vi "Waveform Amplitude Test.vi"(4 "EndRecordMask":i32, 6 "InitialRecordMask":i32, 8 "Lower Constant":dbl, 9 "Upper Constant":dbl=0.001, 10 "Channels to Exclude":string[](array[string]), 11 "Data In":waveform(dbl)[](array[waveform])) -> (1 "Within Limits":bool caption="Passed", 2 "Excluded Channels":waveform(dbl)[](array[waveform]), 3 "Included Channels":waveform(dbl)[](array[waveform]))   [LabVIEW 2019, in "Variant Parser.lvlib" / "WaveformProcessor.lvclass"]
doc: "This routine will look for violations of absolute max and min amplitudes.\nData In: Array of Labview Analog Waveforms to process\nChannels to exclude: Array if channels to ignore testing\nUpper Constant: Upper Amplitude limit\nLower Constant: Lower Amplitude limit\nInitial Record Mask - ignore number of records from t0\nFinal record mask - ignore number of data points from tf"
uses:
  Library/WaveformProcessor.lvclass
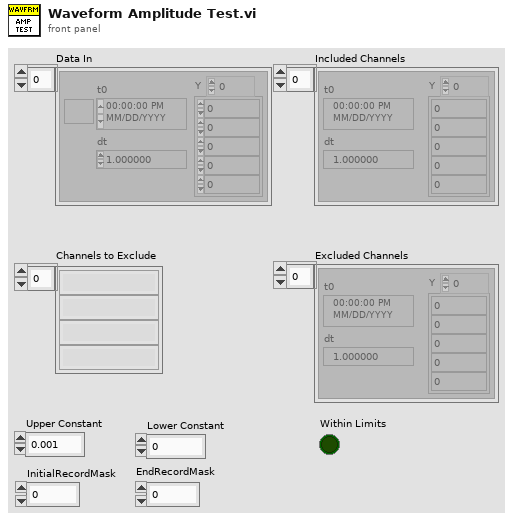
[diagram p1: front panel]
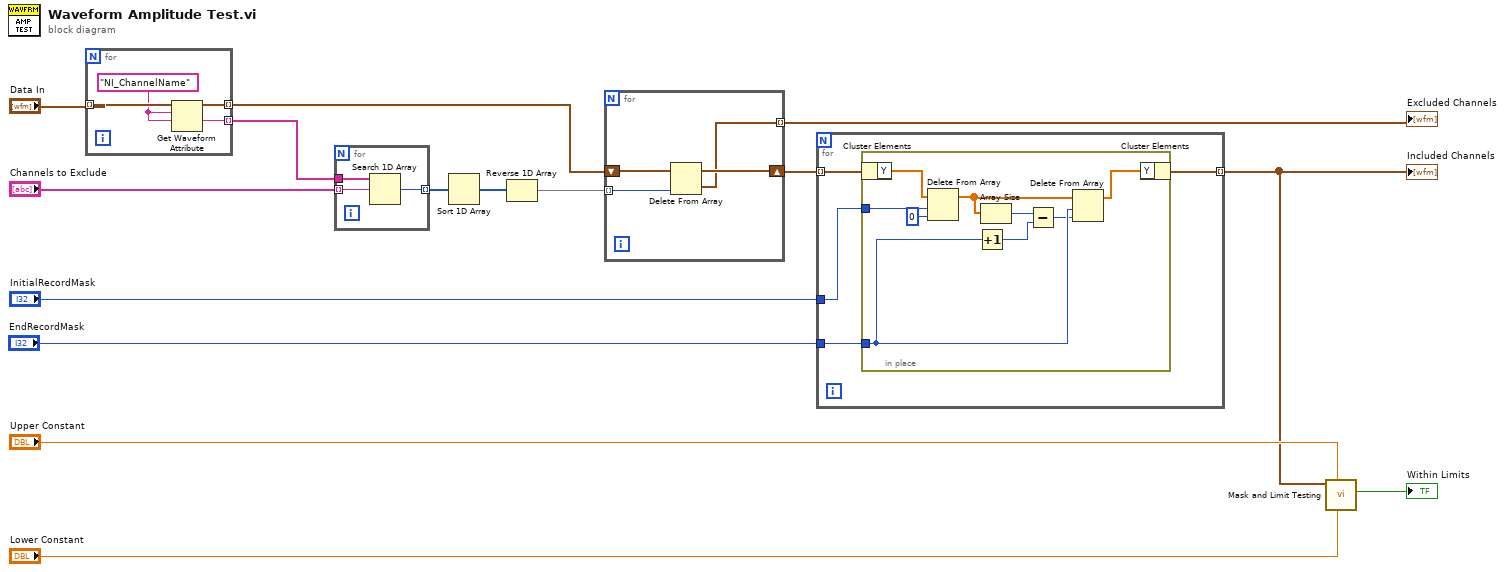
[diagram p0: block diagram]
diagram:
  n1 = for {
    tunnel: [w17] -> w14 mode=indexing
    tunnel: [w16] -> w10 mode=indexing
    tunnel: "Data In" -> [w19] mode=indexing
    w18 = "NI_ChannelName" ("name")
    n2 = Get Waveform Attribute(5:w18, 6:w18, 7:w19) -> (1:w16:string, 3:w17:waveform(dbl))  [unwired: 1 in, 2 out]
  }
  n3 = for {
    tunnel: "Channels to Exclude" -> [w22] mode=indexing
    tunnel: w10 -> [w21]
    tunnel: [w20] -> w11 mode=indexing
    n4 = Search 1D Array(1D array=w21, element=w22) -> (index of element=w20:i32)  [unwired: 1 in]
  }
  n5 = Sort 1D Array(array=w11) -> (sorted array=w12:i32[])
  n6 = Reverse 1D Array(array=w12) -> (reversed array=w13:i32[])
  n7 = for {
    tunnel: w13 -> [w24] mode=indexing
    shift-right: [w25] -> w4
    shift-left: w14 -> [w26]
    tunnel: [w23] -> w15 mode=indexing
    n8 = Delete From Array(array=w26, index=w24) -> (deleted portion=w23:waveform(dbl), array with subset deleted=w25:waveform(dbl)[])  [unwired: 1 in]
  }
  "Excluded Channels" <- w15
  n9 = for {
    tunnel: w4 -> [w30] mode=indexing
    tunnel: [w29] -> w3 mode=indexing
    tunnel: "InitialRecordMask" -> [w28]
    tunnel: "EndRecordMask" -> [w27]
    n10 = in-place {
      in-place-border: w28 -> [w34]
      in-place-border: w27 -> [w32]
      n11 = in-place-cluster #1(w30) -> ("Y"=w39:dbl[])
      n12 = Delete From Array(array=w39, length=w34, index=0) -> (array with subset deleted=w37:dbl[])  [unwired: 1 out]
      n13 = Increment(x=w32) -> (x+1=w33:i32)
      n14 = Array Size(array=w37) -> (size(s)=w36:i32)
      n15 = Subtract(x=w36, y=w33) -> (x-y=w31:i32)
      n16 = Delete From Array(array=w37, length=w32, index=w31) -> (array with subset deleted=w35:dbl[])  [unwired: 1 out]
      n17 = in-place-cluster #1("Y"=w35) -> (w29:waveform(dbl))
    }
  }
  "Included Channels" <- w3
  n18 = call "Mask and Limit Testing"("Lower Constant"="Lower Constant", "Upper Constant"="Upper Constant", "Signals"=w3) -> ("Passed"=→"Within Limits":bool)  [unwired: 5 in, 3 out]
